vi "GetContourResultValue.vi"(11 "ContourResult":T1) -> (3 "ContourResultValue":string[](array[string]))   [LabVIEW 2019]
uses:
  Controls/Contour/Analysis_Contour_Result.ctl
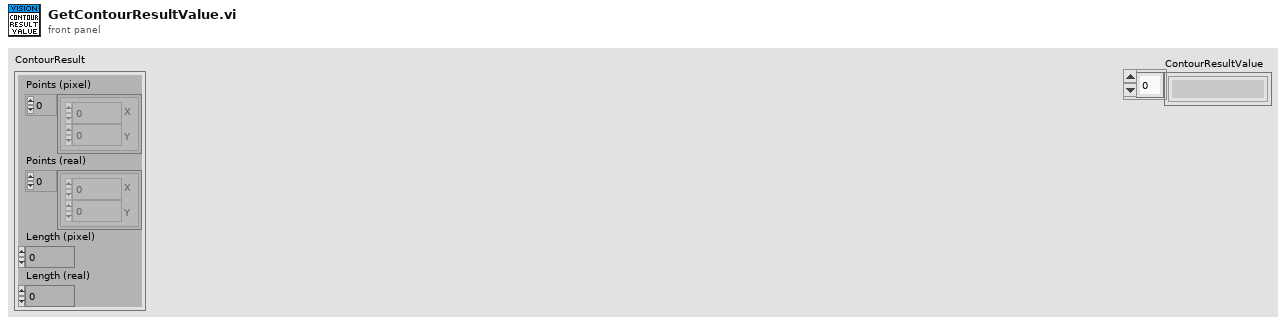
[diagram p1: front panel]
types:
  T1 = typedef "Analysis_Contour_Result.ctl" = cluster{"Points (pixel)":cluster{"X":dbl, "Y":dbl}[], "Points (real)":cluster{"X":dbl, "Y":dbl}[], "Length (pixel)":dbl, "Length (real)":dbl}
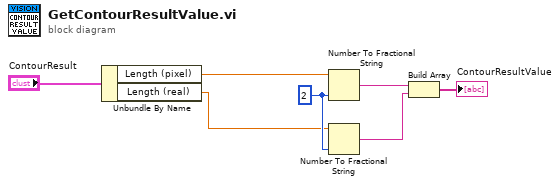
[diagram p0: block diagram]
diagram:
  w5 = i16 2 ("precision (6)")
  n1 = Unbundle By Name("ContourResult") -> ("Length (pixel)"=w6:dbl, "Length (real)"=w4:dbl)
  n2 = Number To Fractional String(number=w6, precision (6)=w5) -> (F-format string=w3:string)  [unwired: 2 in]
  n3 = Number To Fractional String(number=w4, precision (6)=w5) -> (F-format string=w2:string)  [unwired: 2 in]
  n4 = Build Array(w3, w2) -> (→"ContourResultValue":string[])
